vi "Add Network Chassis.vi"(0 "SLSC Local in":refnum<class "SLSC Local.lvclass">, 1 "username":string, 2 "password":string, 5 "chassis IP address/hostname":string, 11 "error in (no error)":errorcluster, 12 "connect timeout (60 sec)":dbl=60.0) -> (4 "SLSC Local out":refnum<class "SLSC Local.lvclass">, 6 "chassis out":refnum<k21>, 15 "error out":errorcluster)   [LabVIEW 2016, in "SLSC Interfaces.lvlib" / "SLSC Local.lvclass"]
uses:
  SLSC Local.lvclass
  C:/Users/tblair/Documents/Git Projects/SLSC-Interface/Source/SLSC Interface Class/SLSC Interface.lvclass
  <vilib>/SLSC/SLSC.lvlib
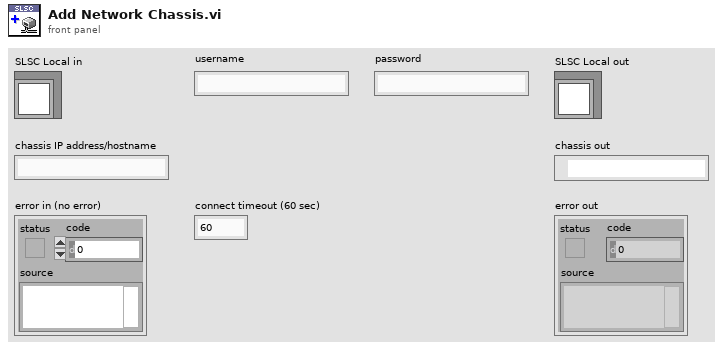
[diagram p1: front panel]
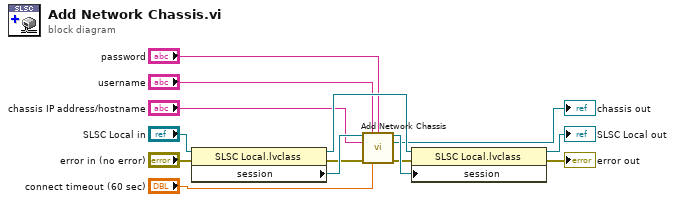
[diagram p0: block diagram]
diagram:
  n1 = property class="SLSC Local.lvclass"(reference="SLSC Local in", error in="error in (no error)") -> (reference out=w14:refnum<class "SLSC Local.lvclass">, error out=w12:errorcluster, "session"=w13:refnum<k21>)
  n2 = call <vilib>:"Add Network Chassis.vi"("session in"=w13, "username"="username", "password"="password", "chassis IP address/hostname"="chassis IP address/hostname", "error in (no error)"=w12, "connect timeout (60 sec)"="connect timeout (60 sec)") -> ("session out"=w11:refnum<k21>, "chassis out"=→"chassis out":refnum<k21>, "error out"=w10:errorcluster)  [unwired: 7 in]
  n3 = property class="SLSC Local.lvclass"(reference=w14, error in=w10, "session"=w11) -> (reference out=→"SLSC Local out":refnum<class "SLSC Local.lvclass">, error out=→"error out":errorcluster)
